vi "AIT 1553 - Parse RT Sysdef Tree Messages.vi"(8 "error in":errorcluster, 9 "RT_Messages":T1[](array[typedef]), 10 "Section Ptr":T3 format="%.0x") -> (0 "error out":errorcluster, 1 "RT_Messages Out":T1[](array[typedef]))   [LabVIEW 2013]
uses:
  <vilib>/NI Veristand/Custom Device API/Custom Device Item Ref.ctl
  Controls/1553_RT_Message.ctl
  Controls/1553 Param.ctl
  Controls and Global/Global.vi
  <vilib>/NI Veristand/Custom Device Tools/Custom Device Utility Library/NI VeriStand - Search for Item by Name.vi
  <vilib>/NI Veristand/Custom Device API/Get Item Property (I32).vi
  <vilib>/NI Veristand/Custom Device API/Get Item Property (Double).vi
  <vilib>/NI Veristand/Custom Device API/Get Item Property (Boolean).vi
  AIT 1553 Custom Device.lvlib
  <vilib>/NI Veristand/Custom Device Tools/Custom Device Utility Library/Custom Device Utility Library.lvlib
  <vilib>/NI Veristand/Custom Device API/Custom Device API.lvlib
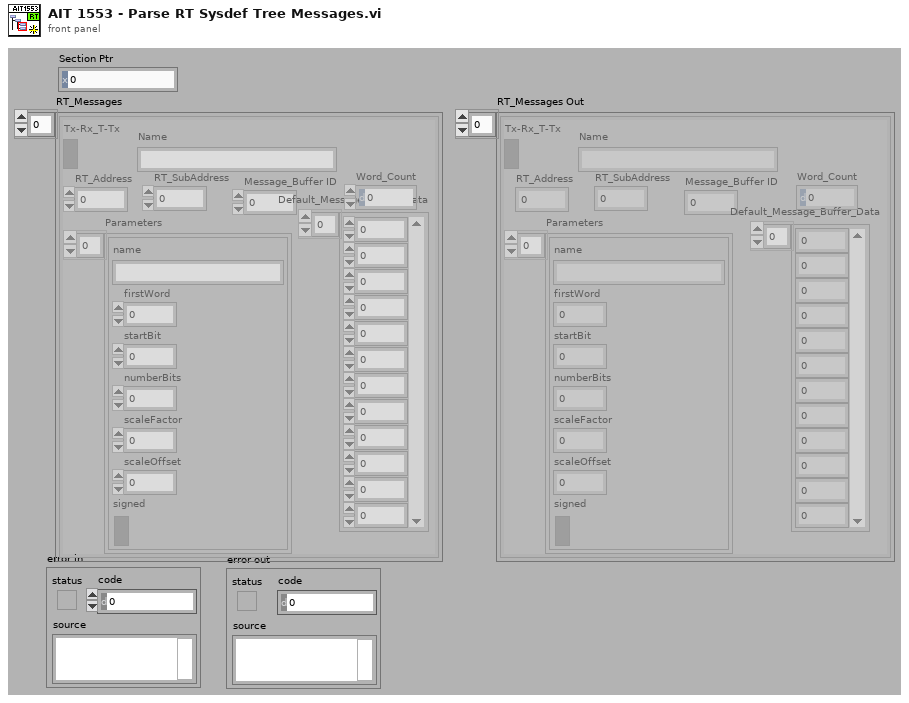
[diagram p1: front panel]
types:
  T1 = typedef "AIT 1553 Custom Device.lvlib/1553_RT_Message.ctl" = cluster{"RT_Address":u8, "RT_SubAddress":u8, "Tx-Rx_T-Tx":bool, "Parameters":T2[], "Message_Buffer ID":u16, "Default_Message_Buffer_Data":u16[], "Word_Count":u8, "Name":string}
  T2 = typedef "AIT 1553 Custom Device.lvlib/1553 Param.ctl" = cluster{"name":string, "firstWord":i32, "startBit":i32, "numberBits":i32, "scaleFactor":dbl, "scaleOffset":dbl, "signed":bool}
  T3 = typedef "Custom Device API.lvlib/Custom Device Item Ref.ctl" = u64
  T4 = typedef "Custom Device API.lvlib/Custom Device Item Info.ctl" = cluster{"Name":string, "Is Channel":bool, "GUID":string, "Is Waveform":bool}
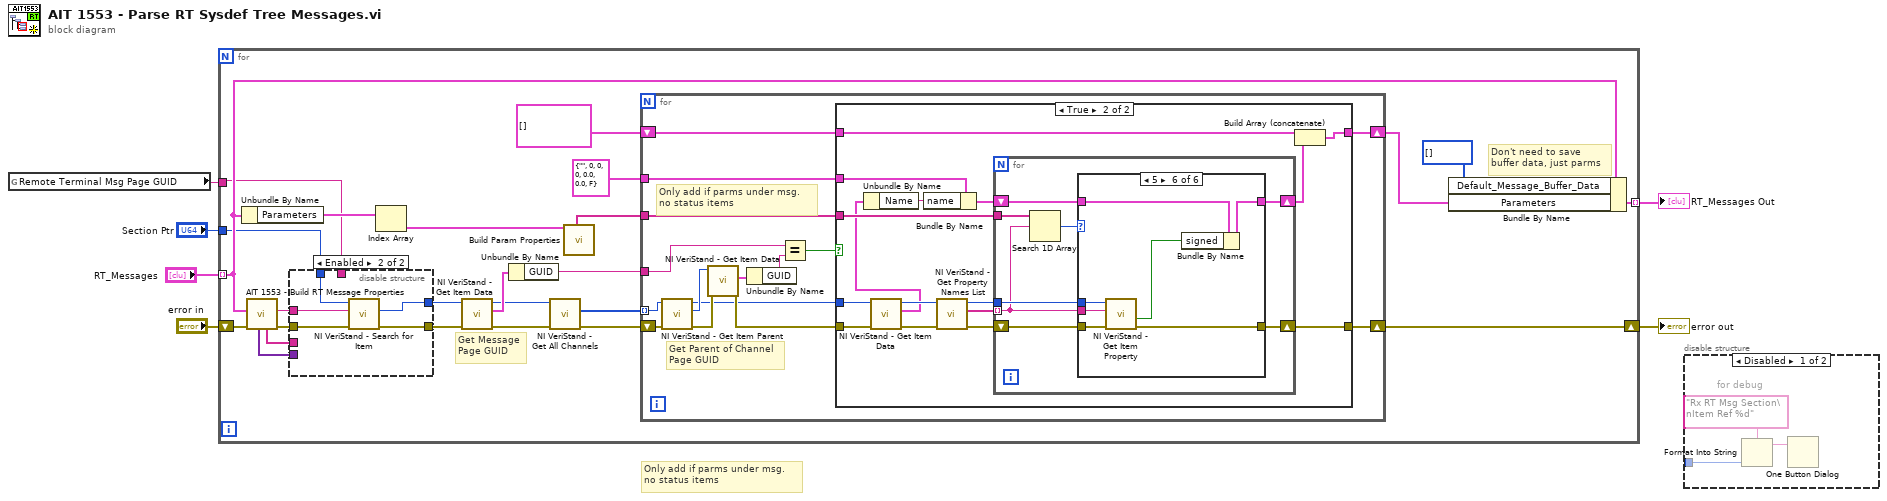
[diagram p0: block diagram]
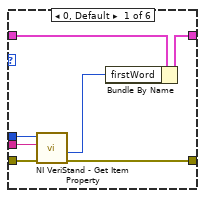
[diagram p4: hidden frame]
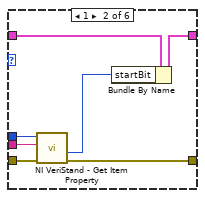
[diagram p5: hidden frame]
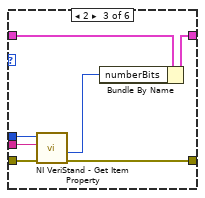
[diagram p6: hidden frame]
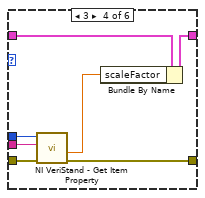
[diagram p7: hidden frame]
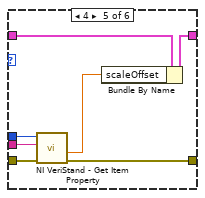
[diagram p8: hidden frame]
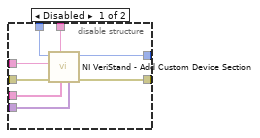
[diagram p9: hidden frame]
diagram:
  # "Only add if parms under msg.\nno status items"
  n1 = global read "Global.vi" "Remote Terminal Msg Page GUID"() -> (w3:string)
  n2 = for {
    shift-right: [w7] -> w6
    shift-left: "error in" -> [w31]
    tunnel: "Section Ptr" -> [w23]
    tunnel: "RT_Messages" -> [w25] mode=indexing
    tunnel: w3 -> [w24]
    tunnel: [w18] -> w1 mode=indexing
    # "Get Message\nPage GUID"
    # "Don't need to save\nbuffer data, just parms"
    n3 = Unbundle By Name(w25) -> ("Parameters"=w28:T2[])
    n4 = call "AIT 1553 - Build RT Message Properties.vi"("error in (no error)"=w31, "RT_Message"=w25) -> ("error out"=w21:errorcluster, "name"=w22:string, "Prop Names"=w20:string[], "Prop Values"=w19:variant[])  [unwired: 5 in, 1 out]
    n5 = disable-structure shown="Enabled" {
      disable-tunnel: w19 -> [w122 _]
      disable-tunnel: w20 -> [w121 _]
      disable-tunnel: w21 -> [w120 w126]
      disable-tunnel: w22 -> [w119 w127]
      disable-tunnel: w24 -> [w118 _]
      disable-tunnel: w23 -> [w117 w125]
      disable-tunnel: [w116 w123] -> w14
      disable-tunnel: [w115 w124] -> w13
      frame Disabled {
        n6 = call <vilib>:"NI VeriStand - Add Custom Device Section.vi"("Property Values"=w122, "Property names"=w121, "GUID (Default Section)"=w118, "error in (no error)"=w120, "Section Name"=w119, "Parent Ref in"=w117) -> ("error out"=w116:errorcluster, "Section Ptr"=w115:T3)  [unwired: 2 in, 2 out]
      }
      frame Enabled {
        n7 = call-poly <vilib>:"NI VeriStand - Search for Item.vi"("error in"=w126, "Item Name"=w127, "Section Ref in"=w125) -> ("error out"=w123:errorcluster, "Item Ref"=w124:T3)  [unwired: 5 in, 2 out]
      }
    }
    n8 = Index Array(array=w28) -> (element=w29:T2)  [unwired: 1 in]
    n9 = call <vilib>:"NI VeriStand - Get Item Data.vi"("error in (no error)"=w14, "Item Ref in"=w13) -> ("error out"=w12:errorcluster, "Item Info"=w15:T4, "Item Ref out"=w11:T3)  [unwired: 6 in, 1 out]
    n10 = Unbundle By Name(w15) -> ("GUID"=w10:string)
    n11 = call <vilib>:"NI VeriStand - Get All Channels.vi"("error in"=w12, "Section Ref in"=w11) -> ("error out"=w26:errorcluster, "Channel Refs"=w27:T3[])  [unwired: 6 in, 2 out]
    n12 = call "Build Param Properties.vi"("1553 Parameter"=w29) -> ("Prop Names"=w30:string[])  [unwired: 10 in, 8 out]
    n13 = for {
      tunnel: w27 -> [w41] mode=indexing
      tunnel: w30 -> [w46]
      tunnel: T2 {"name"="", "firstWord"=0, "startBit"=0, "numberBits"=0, "scaleFactor"=0.0, "scaleOffset"=0.0, "signed"=FALSE} ("1553 Parameter") -> [w44]
      tunnel: w10 -> [w36]
      shift-right: [w32] -> w8
      shift-left: T2[] [] -> [w33]
      shift-right: [w45] -> w7
      shift-left: w26 -> [w40]
      # "Only add if parms under msg.\nno status items"
      # "Get Parent of Channel\nPage GUID"
      n14 = call <vilib>:"NI VeriStand - Get Item Parent.vi"("error in (no error)"=w40, "Item Ref in"=w41) -> ("error out"=w43:errorcluster, "Parent Ref"=w42:T3, "Item Ref out"=w38:T3)  [unwired: 6 in, 1 out]
      n15 = call <vilib>:"NI VeriStand - Get Item Data.vi"("error in (no error)"=w43, "Item Ref in"=w42) -> ("error out"=w39:errorcluster, "Item Info"=w37:T4)  [unwired: 6 in, 2 out]
      n16 = Unbundle By Name(w37) -> ("GUID"=w34:string)
      n17 = Equal?(x=w36, y=w34) -> (x = y?=w35:bool)
      n18 = case shown="True" w35 {
        tunnel: w46 -> [_ w62]
        tunnel: [w47 w49] -> w45
        tunnel: w44 -> [_ w57]
        tunnel: w39 -> [w47 w54]
        tunnel: w38 -> [_ w53]
        tunnel: w33 -> [w48 w52]
        tunnel: [w48 w50] -> w32
        frame False {
        }
        frame True {
          n19 = call <vilib>:"NI VeriStand - Get Item Data.vi"("error in (no error)"=w54, "Item Ref in"=w53) -> ("error out"=w60:errorcluster, "Item Info"=w55:T4, "Item Ref out"=w59:T3)  [unwired: 6 in, 1 out]
          n20 = Unbundle By Name(w55) -> ("Name"=w58:string)
          n21 = Bundle By Name(cluster=w57, "name"=w58) -> (w56:T2)
          n22 = call <vilib>:"NI VeriStand - Get Property Names List.vi"("error in (no error)"=w60, "Item Ref in"=w59) -> ("error out"=w64:errorcluster, "Property Names"=w63:string[], "Item Ref out"=w61:T3)  [unwired: 7 in]
          n23 = for {
            tunnel: w63 -> [w67] mode=indexing
            tunnel: w62 -> [w72]
            shift-right: [w66] -> w51
            shift-left: w56 -> [w70]
            tunnel: w61 -> [w68]
            shift-right: [w65] -> w49
            shift-left: w64 -> [w69]
            n24 = Search 1D Array(1D array=w72, element=w67) -> (index of element=w71:i32)  [unwired: 1 in]
            n25 = case shown="5" w71 {
              tunnel: w70 -> [w79 w86 w93 w100 w107 w114]
              tunnel: w69 -> [w78 w85 w92 w99 w106 w113]
              tunnel: w68 -> [w77 w84 w91 w98 w105 w112]
              tunnel: w67 -> [w76 w83 w90 w97 w104 w111]
              tunnel: [w74 w81 w88 w95 w102 w109] -> w66
              tunnel: [w73 w80 w87 w94 w101 w108] -> w65
              frame 0, Default {
                n26 = call-poly <vilib>:"NI VeriStand - Get Item Property.vi"("error in (no error)"=w78, "Property Name"=w76, "Item Ref in"=w77) -> ("error out"=w73:errorcluster, "Value"=w75:i32)  [unwired: 5 in, 2 out]
                n27 = Bundle By Name(cluster=w79, "firstWord"=w75) -> (w74:T2)
              }
              frame 1 {
                n28 = call-poly <vilib>:"NI VeriStand - Get Item Property.vi"("error in (no error)"=w85, "Property Name"=w83, "Item Ref in"=w84) -> ("error out"=w80:errorcluster, "Value"=w82:i32)  [unwired: 5 in, 2 out]
                n29 = Bundle By Name(cluster=w86, "startBit"=w82) -> (w81:T2)
              }
              frame 2 {
                n30 = call-poly <vilib>:"NI VeriStand - Get Item Property.vi"("error in (no error)"=w92, "Property Name"=w90, "Item Ref in"=w91) -> ("error out"=w87:errorcluster, "Value"=w89:i32)  [unwired: 5 in, 2 out]
                n31 = Bundle By Name(cluster=w93, "numberBits"=w89) -> (w88:T2)
              }
              frame 3 {
                n32 = call-poly <vilib>:"NI VeriStand - Get Item Property.vi"("error in (no error)"=w99, "Property Name"=w97, "Item Ref in"=w98) -> ("error out"=w94:errorcluster, "Value"=w96:dbl)  [unwired: 5 in, 2 out]
                n33 = Bundle By Name(cluster=w100, "scaleFactor"=w96) -> (w95:T2)
              }
              frame 4 {
                n34 = call-poly <vilib>:"NI VeriStand - Get Item Property.vi"("error in (no error)"=w106, "Property Name"=w104, "Item Ref in"=w105) -> ("error out"=w101:errorcluster, "Value"=w103:dbl)  [unwired: 5 in, 2 out]
                n35 = Bundle By Name(cluster=w107, "scaleOffset"=w103) -> (w102:T2)
              }
              frame 5 {
                n36 = call-poly <vilib>:"NI VeriStand - Get Item Property.vi"("error in (no error)"=w113, "Property Name"=w111, "Item Ref in"=w112) -> ("error out"=w108:errorcluster, "Value"=w110:bool)  [unwired: 5 in, 2 out]
                n37 = Bundle By Name(cluster=w114, "signed"=w110) -> (w109:T2)
              }
            }
          }
          n38 = Build Array (concatenate)(w52, w51) -> (w50:T2[])
        }
      }
    }
    n39 = Bundle By Name(cluster=w25, "Default_Message_Buffer_Data"=u16[] [], "Parameters"=w8) -> (w18:T1)
  }
  "error out" <- w6
  "RT_Messages Out" <- w1
  n40 = disable-structure shown="Disabled" {
    disable-tunnel: _ -> [w128 _]
    frame Disabled {
      # "for debug"
      n41 = Format Into String(format string="Rx RT Msg Section\nItem Ref %d" ("message"), w128) -> (resulting string=w130:string)  [unwired: 2 in, 1 out]
      n42 = One Button Dialog(message=w130) -> ()  [unwired: 1 in, 1 out]
    }
    frame Enabled {
    }
  }
